vi "DATA out.vi"(7 "Class in":refnum<class "Retrieved Data.lvclass">) -> (2 "Data":T1, 3 "Class Out":refnum<class "Retrieved Data.lvclass">)   [LabVIEW 2017, in "Retrieved Data.lvclass"]
uses:
  Retrieved Data.lvclass
  Retrieved Data.lvclass/Retrieved Data.ctl
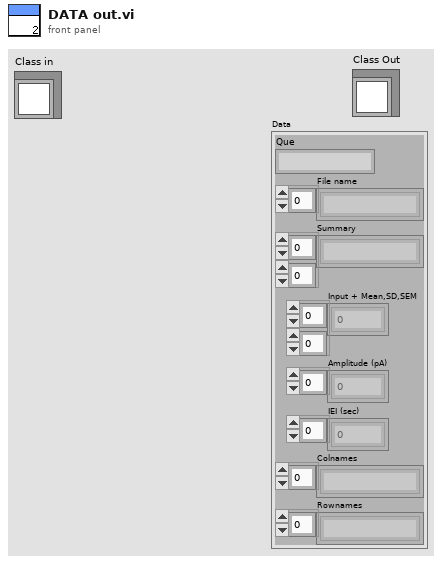
[diagram p1: front panel]
types:
  T1 = cluster{"Que":string, "File name":string[], "Summary":string[][], "Input + Mean,SD,SEM":dbl[][], "Amplitude (pA)":dbl[], "IEI (sec)":dbl[], "Colnames":string[], "Rownames":string[]}
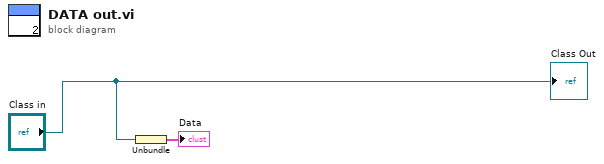
[diagram p0: block diagram]
diagram:
  n1 = Unbundle("Class in") -> (→"Data":T1)
  "Class Out" <- "Class in"
